vi "clear_buffers.vi"(8 "error in (no error)":errorcluster, 11 "FPGAWrapperDL090211Galvo in":refnum<class "FPGAWrapperDL090211Galvo.lvclass">) -> (0 "error out":errorcluster, 3 "FPGAWrapperDL090211Galvo out":refnum<class "FPGAWrapperDL090211Galvo.lvclass">)   [LabVIEW 2010, in "FPGAWrapperDL090211Galvo.lvclass"]
uses:
  FPGAWrapperDL090211Galvo.lvclass
  <vilib>/rvi/interface/nirviMethod/nirviMethod.xnode
  FPGA_VI_ref.ctl
  <vilib>/Utility/error.llb/Error Cluster From Error Code.vi
  NiFpgaLv.dll
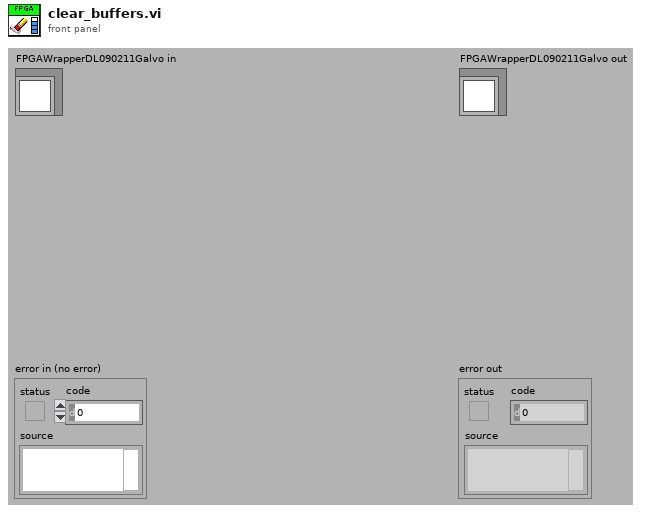
[diagram p1: front panel]
types:
  T1 = typedef "FPGAWrapperDL090211Galvo.lvclass/FPGA_VI_ref.ctl" = refnum<k20>
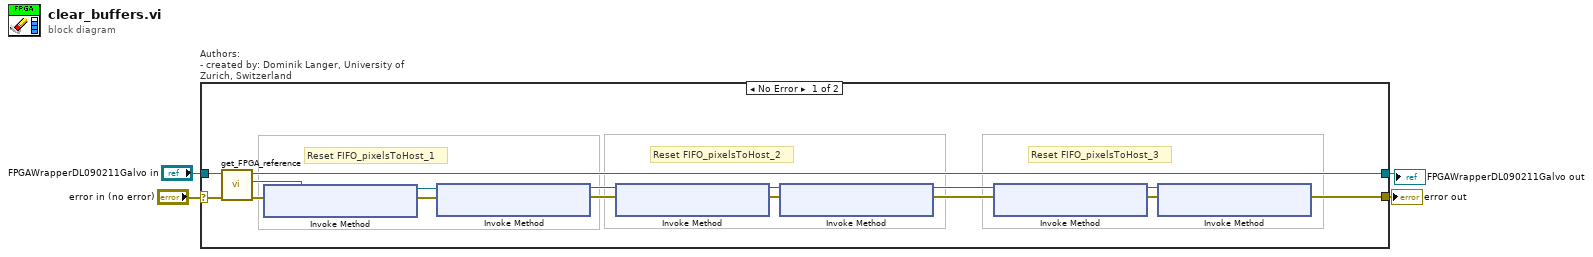
[diagram p0: block diagram]
diagram:
  n1 = case "Authors: \n- created by: Dominik Langer, University of Zurich, Switzerland" shown="No Error" "error in (no error)" {
    selector: "error in (no error)" -> [w20 w153]
    tunnel: "FPGAWrapperDL090211Galvo in" -> [w19 w154]
    tunnel: [w16 w154] -> w2
    tunnel: [w5 w153] -> w1
    frame No Error {
      # "Reset FIFO_pixelsToHost_3"
      # "Reset FIFO_pixelsToHost_2"
      # "Reset FIFO_pixelsToHost_1"
      n2 = call-dynamic "get_FPGA_reference.vi"("error in (no error)"=w20, "FPGAWrapperDL090211Galvo in"=w19) -> ("error out"=w17:errorcluster, "FPGA VI reference"=w18:T1, "FPGAWrapperDL090211Galvo out"=w16:refnum<class "FPGAWrapperDL090211Galvo.lvclass">)  [unwired: 6 in, 1 out]
      n3 = xnode "Invoke Method"("FPGA VI Reference In"=w18, "error in"=w17) -> ("FPGA VI Reference Out"=w15:T1, "error out"=w14:errorcluster)
      n4 = xnode "Invoke Method"("FPGA VI Reference In"=w15, "error in"=w14) -> ("FPGA VI Reference Out"=w13:T1, "error out"=w12:errorcluster)
      n5 = xnode "Invoke Method"("FPGA VI Reference In"=w13, "error in"=w12) -> ("FPGA VI Reference Out"=w11:T1, "error out"=w10:errorcluster)
      n6 = xnode "Invoke Method"("FPGA VI Reference In"=w11, "error in"=w10) -> ("FPGA VI Reference Out"=w7:T1, "error out"=w6:errorcluster)
      n7 = xnode "Invoke Method"("FPGA VI Reference In"=w7, "error in"=w6) -> ("FPGA VI Reference Out"=w9:T1, "error out"=w8:errorcluster)
      n8 = xnode "Invoke Method"("FPGA VI Reference In"=w9, "error in"=w8) -> ("error out"=w5:errorcluster)  [unwired: 1 out]
    }
    frame Error {
    }
  }
  "error out" <- w1
  "FPGAWrapperDL090211Galvo out" <- w2
